vi "TrajCheck.vi"(1 "TrajIn":dbl[][](array[numeric])) -> (0 "GoodTrajectory?":bool)   [LabVIEW 2016, in "ForceField.lvclass"]
uses:
  ForceField.lvclass
panel:
  in  "DistBwTrajEnd":dbl=0.1
  in  "GaitLengthMax":dbl=1.5
  in  "GaitHeightMax":dbl=0.5
  out "TrajOut":dbl[][](array[numeric])
  in  "GaitLengthMin":dbl=0.3
  in  "GaitHeightMin":dbl=0.1
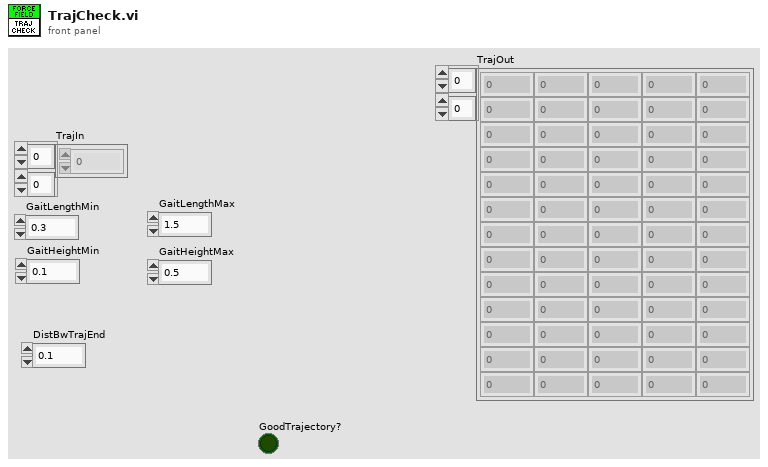
[diagram p1: front panel]
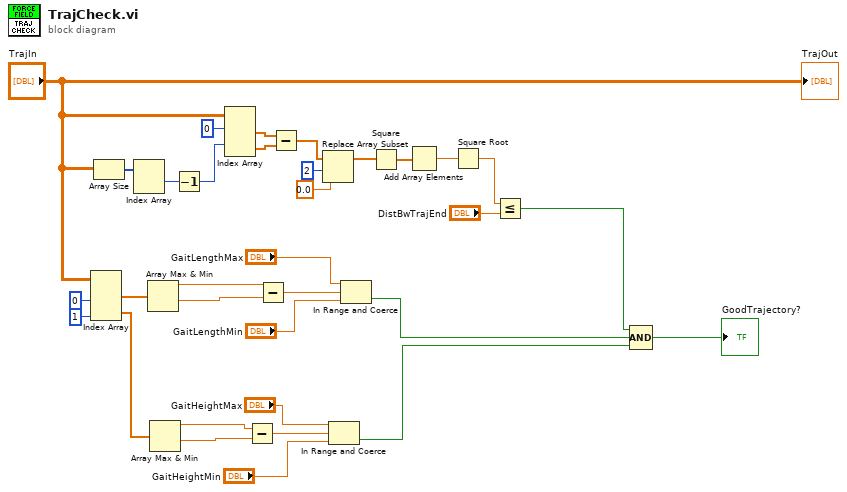
[diagram p0: block diagram]
diagram:
  n1 = Index Array(array="TrajIn", index (col) #1=0 ("index (row)"), index (col) #2=1 ("index (row)")) -> (element #1=w27:dbl[], element #2=w28:dbl[])  [unwired: 2 in]
  n2 = Array Size(array="TrajIn") -> (size(s)=w17:i32[])
  n3 = Index Array(array=w17) -> (element #1=w1:i32)  [unwired: 2 in, 1 out]
  n4 = Array Max & Min(array=w27) -> (max value=w29:dbl, min value=w30:dbl)  [unwired: 2 out]
  n5 = Array Max & Min(array=w28) -> (max value=w31:dbl, min value=w32:dbl)  [unwired: 2 out]
  n6 = Decrement(x=w1) -> (x-1=w4:i32)
  n7 = Index Array(array="TrajIn", index (row) #1=0 ("disabled index (col)"), index (row) #2=w4) -> (element #1=w16:dbl[], element #2=w15:dbl[])  [unwired: 2 in]
  n8 = Subtract(x=w31, y=w32) -> (x-y=w24:dbl)
  n9 = Subtract(x=w29, y=w30) -> (x-y=w26:dbl)
  n10 = Subtract(x=w16, y=w15) -> (x-y=w14:dbl[])
  n11 = Replace Array Subset(array=w14, new element=0.0 ("new element/subarray"), index=2) -> (w11:dbl[])
  n12 = In Range and Coerce(upper limit="GaitHeightMax", x=w24, lower limit="GaitHeightMin") -> (In Range?=w19:bool)  [unwired: 1 out]
  n13 = In Range and Coerce(upper limit="GaitLengthMax", x=w26, lower limit="GaitLengthMin") -> (In Range?=w20:bool)  [unwired: 1 out]
  n14 = Square(x=w11) -> (x^2=w10:dbl[])
  n15 = Add Array Elements(numeric array=w10) -> (sum=w9:dbl)
  n16 = Square Root(x=w9) -> (sqrt(x)=w8:dbl)
  n17 = Less Or Equal?(x=w8, y="DistBwTrajEnd") -> (x <= y?=w6:bool)
  n18 = Compound Arithmetic op=AND(w6, w20, w19) -> (→"GoodTrajectory?":bool)
  "TrajOut" <- "TrajIn"
